vi "XIPIN_AXI_DataMover_5_1.vi"   [LabVIEW 2017]
doc: "AXI DataMover is a soft Xilinx IP core used as a building block for scalable DMA functions. It provides the basic AXI4 Memory Map Read to AXI4-Stream and AXI4-Stream to AXI4 Memory Map Write data transport and protocol conversion. It supports Synchronous/Asynchronous clocking for Command/Status interface. Supports Memory Map and Stream side data widht up to 1024 bits and Memory Map address width up to 64-bit. AXI Datamover core also provide optional Data Realignment Engine (DRE) upto 64-bit of stream data width, General purpose Store and Forward unit, Interminate BTT mode.\n------------------------------------\n<b>Need License</b> : No\n<b>Interface</b> : AXI4 AXI4-Stream"
uses:
  <vilib>/rvi/XilinxIP/XIPIN_XNode/niFpgaXIPIN.xnode
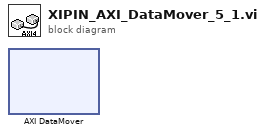
[diagram p0: block diagram]
diagram:
  n1 = xnode ("AXI DataMover")() -> ()
